vi "element_editor.vi"(4 "Break":refnum<vi>, 5 "LUA Specification File":path) -> (0 "Cancelled?":bool)   [LabVIEW 2019]
panel:
  in  "Save As Button":bool
  out "Validation":string
  out "ButtonCluster":T1
  in  "Cancel Button":bool
  in  "Save Button":bool
  out "Vali File Loaded":bool
  in  "Load Vali File":bool
  in  "Load Validation File":path
  in  "Validate":bool
  in  "Parameters":string(tree)="_3"
  # "Biogas Editor"
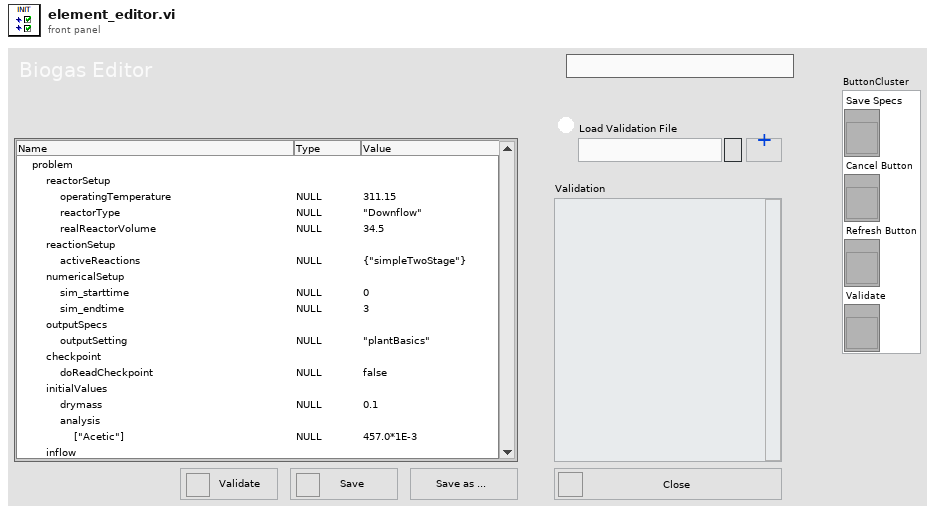
[diagram p1: front panel]
types:
  T1 = cluster{"Save Specs":refnum<vi>, "Cancel Button":refnum<vi>, "Refresh Button":refnum<vi>, "Validate":refnum<vi>}
  T2 = cluster{"Save Button":refnum<vi>, "Cancel Button":refnum<vi>, "Save As Button ":refnum<vi>, "Validate":refnum<vi>}
  T3 = enum8{"Enabled", "Disabled", "Disabled and Grayed Out"}
  T4 = typedef "LVPoint32TypeDef.ctl" = cluster{"Horizontal":i32, "Vertical":i32}
  T5 = enum32{"Invalid", "Standard", "Closed", "Hidden", "Minimized", "Maximized"}
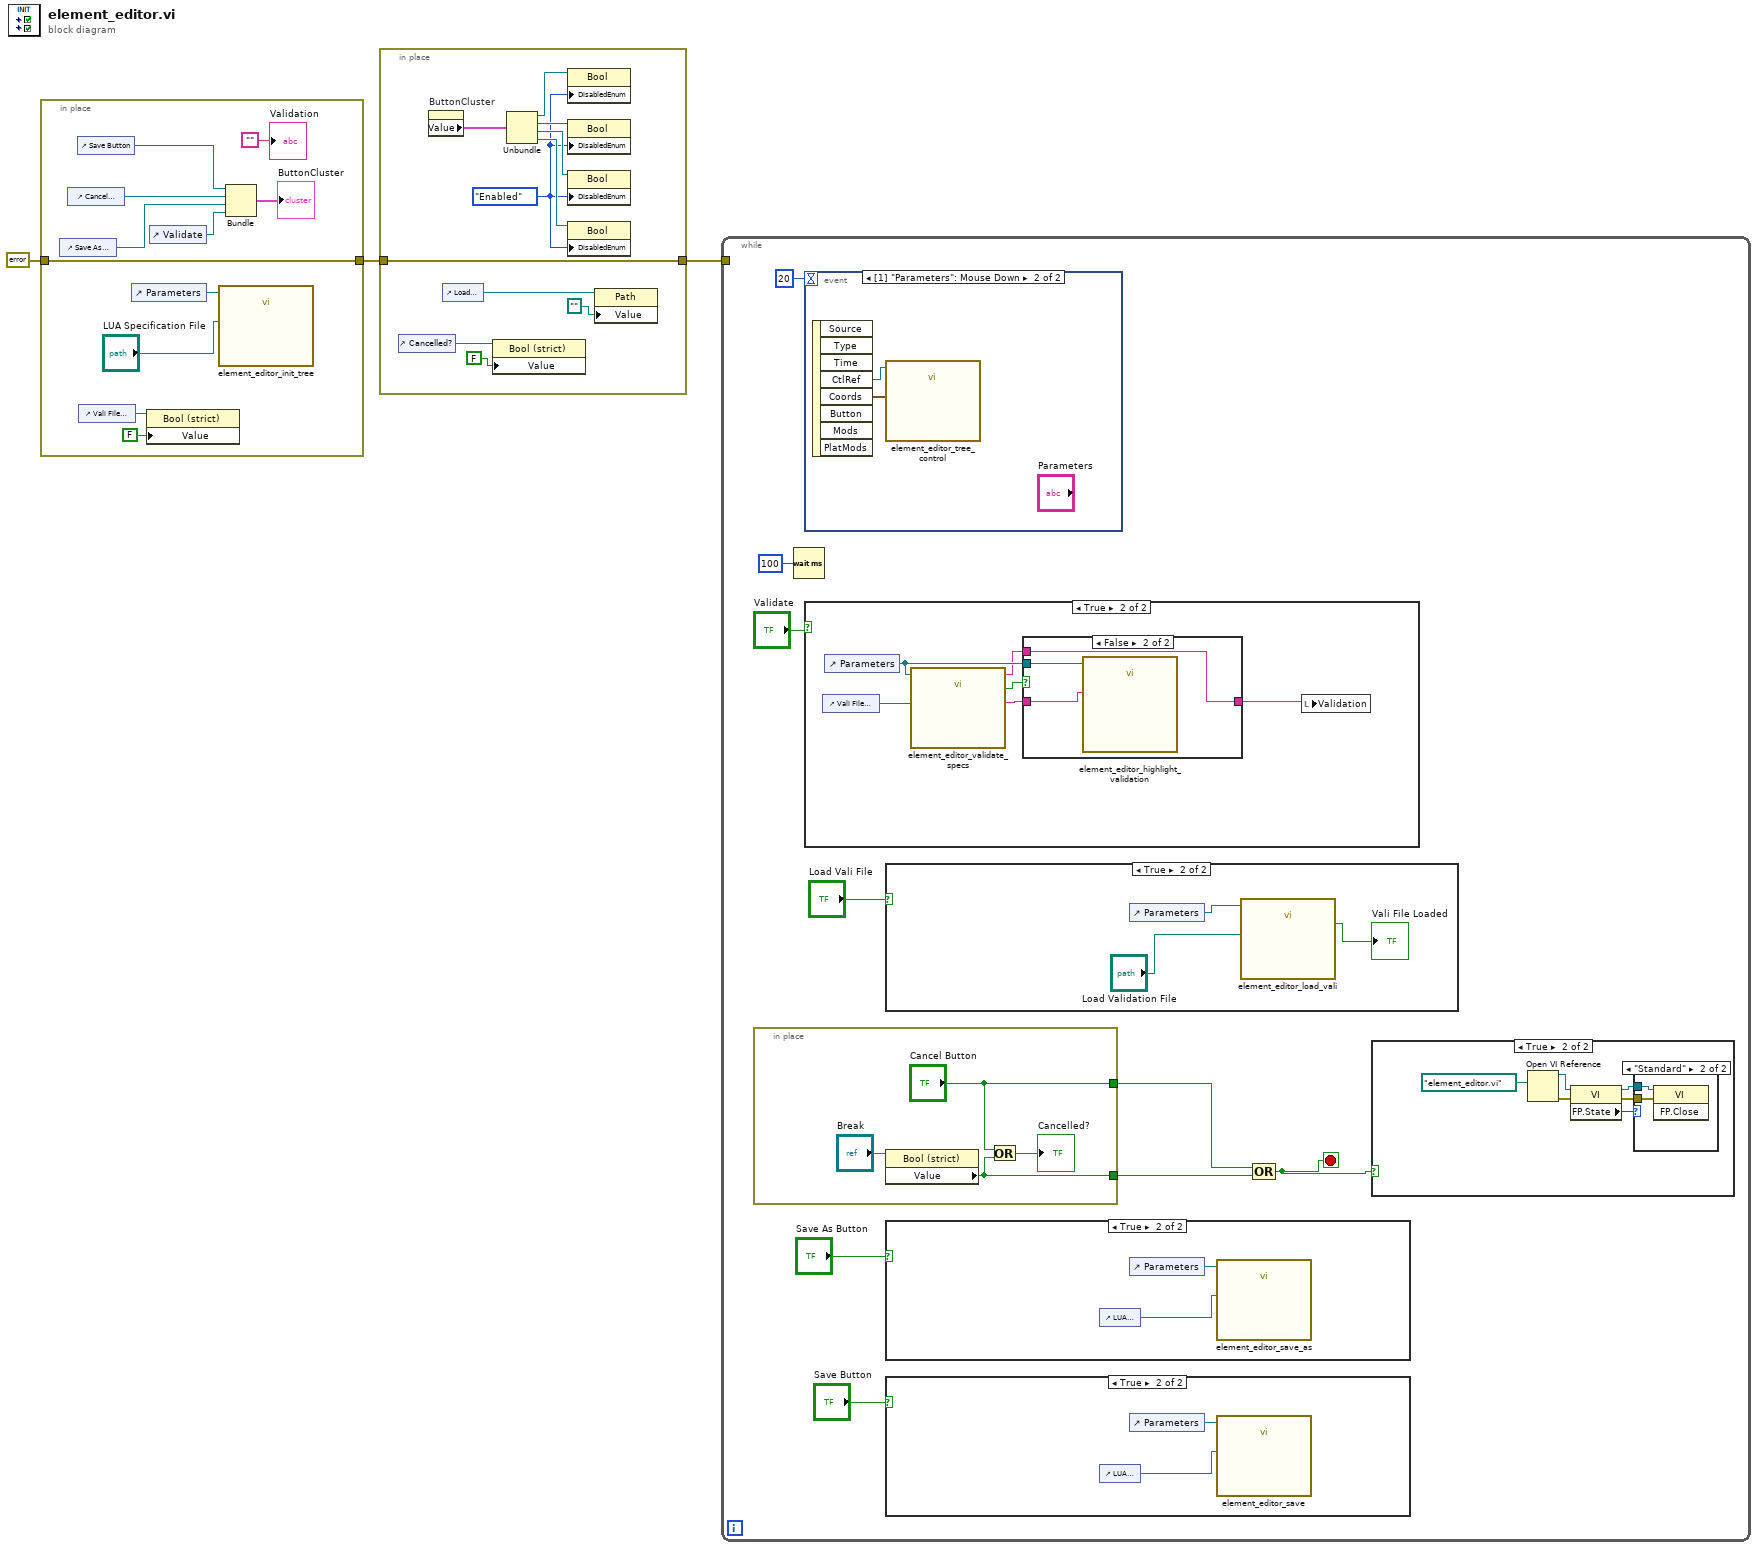
[diagram p0: block diagram]
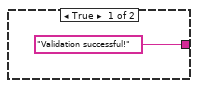
[diagram p7: hidden frame]
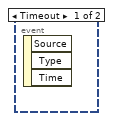
[diagram p9: hidden frame]
diagram:
  n1 = in-place {
    in-place-border: errorcluster {"status"=FALSE, "code"=0, "source"=""} ("error constant") -> [w14]
    in-place-border: [w14] -> w2
    n2 = control-ref of="Save As Button"() -> (w7:refnum<vi>)
    n3 = control-ref of="Cancel Button"() -> (w12:refnum<vi>)
    n4 = control-ref of="Save Button"() -> (w11:refnum<vi>)
    n5 = control-ref of="Vali File Loaded"() -> (w6:refnum<vi>)
    n6 = control-ref of="Parameters"() -> (w9:refnum<vi>)
    n7 = property class="Bool (strict)"(reference=w6, "Value"=FALSE) -> ()  [unwired: 1 in, 2 out]
    n8 = control-ref of="Validate"() -> (w13:refnum<vi>)
    n9 = call "element_editor_init_tree.vi"("LUA Specification File"="LUA Specification File", "TreeControl in"=w9) -> ()  [unwired: 10 in]
    n10 = Bundle("Save Button"=w11, "Cancel Button"=w12, "Save As Button"=w7, "Validate"=w13) -> (→"ButtonCluster":T2)  [unwired: 1 in]
    "Validation" <- ""
  }
  n11 = in-place {
    in-place-border: [w25] -> w1
    in-place-border: w2 -> [w25]
    w15 = T3."Enabled" ("Disabled")
    n12 = control-ref of="Cancelled?"() -> (w24:refnum<vi>)
    n13 = property on="ButtonCluster" class="Clust (strict)"() -> ("Value"=w19:T1)  [unwired: 2 in, 2 out]
    n14 = control-ref of="Load Validation File"() -> (w23:refnum<vi>)
    n15 = property on="Property Node" class="Bool (strict)"(reference=w24, "Value"=FALSE ("Stop Button")) -> ()  [unwired: 1 in, 2 out]
    n16 = Unbundle(w19) -> ("Save Specs"=w22:refnum<vi>, "Cancel Button"=w21:refnum<vi>, "Refresh Button"=w16:refnum<vi>, "Validate"=w20:refnum<vi>)
    n17 = property on="Property Node" class="Bool"(reference=w22, "DisabledEnum"=w15) -> ()  [unwired: 1 in, 2 out]
    n18 = property on="Property Node" class="Bool"(reference=w21, "DisabledEnum"=w15) -> ()  [unwired: 1 in, 2 out]
    n19 = property on="Property Node" class="Bool"(reference=w16, "DisabledEnum"=w15) -> ()  [unwired: 1 in, 2 out]
    n20 = property on="Property Node" class="Bool"(reference=w20, "DisabledEnum"=w15) -> ()  [unwired: 1 in, 2 out]
    n21 = property class="Path"(reference=w23, "Value"=path "") -> ()  [unwired: 1 in, 2 out]
  }
  n22 = while {
    tunnel: w1 -> [_]
    stop <- w29 stop-if-true
    n23 = in-place {
      in-place-border: ["Cancel Button"] -> w28
      in-place-border: [w45] -> w27
      n24 = property class="Bool (strict)"(reference="Break") -> ("Value"=w45:bool)  [unwired: 1 in, 2 out]
      n25 = Or(x="Cancel Button", y=w45) -> (x .or. y?=→"Cancelled?":bool)
    }
    n26 = Wait (ms)(milliseconds to wait=u32 100) -> ()  [unwired: 1 out]
    n27 = event shown="[1] \"Parameters\": Mouse Down" {
      selector: _ -> [_ _]
      dyn-events: _ -> [_ _]
      timeout: 20 -> [_ _]
      event Timeout {
        n28 = event-data() -> ()  [unwired: 1 in, 3 out]
      }
      event "Parameters": Mouse Down {
        n29 = event-data() -> ("CtlRef"=w64:refnum<vi>, "Coords"=w65:T4)  [unwired: 1 in, 6 out]
        n30 = call "element_editor_tree_control.vi"("Point"=w65, "Parameters Tree"=w64) -> ()  [unwired: 10 in]
      }
    }
    n31 = case shown="True" "Validate" {
      frame False {
      }
      frame True {
        n32 = control-ref of="Vali File Loaded"() -> (w54:refnum<vi>)
        n33 = control-ref of="Parameters"() -> (w55:refnum<vi>)
        n34 = call "element_editor_validate_specs.vi"("Vali File Loaded?"=w54, "Parameters Tree"=w55) -> ("validationErrors"=w56:string, "Valid?"=w53:bool, "validationMsg"=w51:string)  [unwired: 7 in]
        n35 = case shown="False" w53 {
          tunnel: w56 -> [_ w60]
          tunnel: w55 -> [_ w59]
          tunnel: ["Validation successful!" ("message") w58] -> w52
          tunnel: w51 -> [_ w58]
          frame True {
          }
          frame False {
            n36 = call "element_editor_highlight_validation.vi"("validationErrors"=w60, "Parameters Tree"=w59) -> ()  [unwired: 10 in]
          }
        }
        n37 = local write "Validation"(w52) -> ()
      }
    }
    n38 = case shown="True" "Load Vali File" {
      frame False {
      }
      frame True {
        n39 = control-ref of="Parameters"() -> (w62:refnum<vi>)
        n40 = call "element_editor_load_vali.vi"("LUA Validation File"="Load Validation File", "Parameters Tree"=w62) -> ("Vali File Loaded"=→"Vali File Loaded":bool)  [unwired: 9 in]
      }
    }
    n41 = case shown="True" "Save As Button" {
      frame False {
      }
      frame True {
        n42 = control-ref of="LUA Specification File"() -> (w36:refnum<vi>)
        n43 = control-ref of="Parameters"() -> (w35:refnum<vi>)
        n44 = call "element_editor_save_as.vi"("Specification Path"=w36, "Parameters Tree"=w35) -> ()  [unwired: 10 in]
      }
    }
    n45 = case shown="True" "Save Button" {
      frame False {
      }
      frame True {
        n46 = control-ref of="LUA Specification File"() -> (w49:refnum<vi>)
        n47 = control-ref of="Parameters"() -> (w50:refnum<vi>)
        n48 = call "element_editor_save.vi"("Specification Path"=w49, "Parameters Tree"=w50) -> ()  [unwired: 10 in]
      }
    }
    n49 = Compound Arithmetic op=OR(w28, w27) -> (w29:bool)
    n50 = case shown="True" w29 {
      frame False {
      }
      frame True {
        n51 = Open VI Reference(vi path=path "element_editor.vi") -> (vi reference=w38:refnum<vi>, error out=w37:errorcluster)  [unwired: 5 in]
        n52 = property class="VI"(reference=w38, error in=w37) -> (reference out=w40:refnum<vi>, error out=w39:errorcluster, "FP.State"=w41:T5)
        n53 = case shown="\"Standard\"" w41 {
          tunnel: w40 -> [_ w44]
          tunnel: w39 -> [_ w43]
          frame "Invalid", Default {
          }
          frame "Standard" {
            n54 = invoke class="VI" method="FP.Close"(reference=w44, error in=w43) -> ()  [unwired: 1 in, 3 out]
          }
        }
      }
    }
  }
